vi "Deep Copy.vi"(7 "Tree ID":string, 8 "Error In":errorcluster, 11 "Tree Manager":T1) -> (0 "Error Out":errorcluster, 3 "Tree Manager":T1, 5 "Unique ID of Copied Tree":string)   [LabVIEW 2020, in "NI_VIAnCFGDataStructure.lvlib" / "Tree.lvclass"]
doc: "Deep copy of a Tree and its attributes. Copies the Children of the Tree all the way down. On all attributes that are Tree Data types a Copy method is invoked. Overwrite the Copy the method in child types of Tree Data to implement special copying mechanism. The Default mechanism is copying by values i.e. LV fork.\n\n<b>WARNING</b> Running this method on a big tree might result in a significantly slower operation than Shallow Copy method. Make sure you need to copy all the Children. If not use Shallow Copy method."
uses:
  <vilib>/addons/analyzer/VIAnCFGDataStructure/Tree Manager/Tree.lvclass
  <vilib>/addons/analyzer/VIAnCFGDataStructure/Tree Manager/Typedefs/Session Handle.ctl
  <vilib>/addons/analyzer/VIAnCFGDataStructure/Tree Manager/Tree.lvclass/Tree.ctl
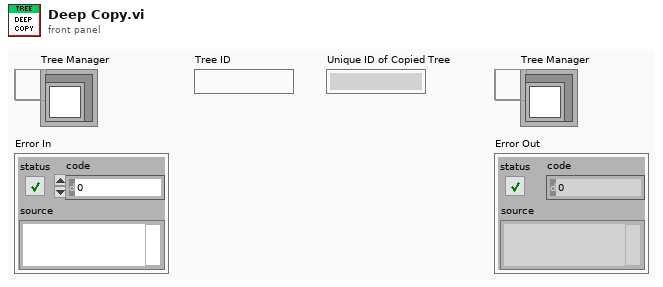
[diagram p1: front panel]
types:
  T1 = typedef "NI_VIAnCFGDataStructure.lvlib/Tree.lvclass/Session Handle.ctl" = refnum<data-value>
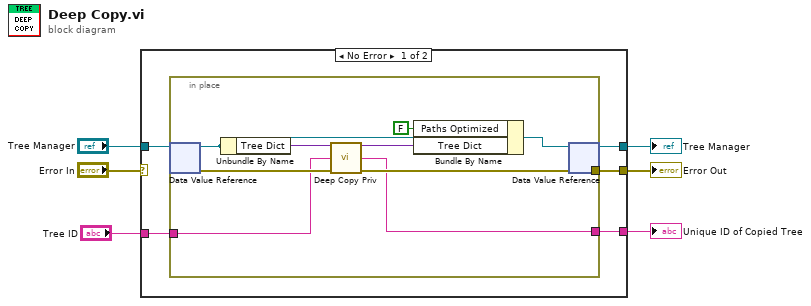
[diagram p0: block diagram]
diagram:
  n1 = case shown="No Error" "Error In" {
    selector: "Error In" -> [_ w21]
    tunnel: "Tree Manager" -> [w11 w22]
    tunnel: [w10 w22] -> w5
    tunnel: [w9 w21] -> w3
    tunnel: "Tree ID" -> [w8 _]
    tunnel: [w7 _] -> w1
    frame No Error {
      n2 = in-place {
        in-place-border: [w19] -> w9
        in-place-border: w8 -> [w16]
        in-place-border: [w15] -> w7
        n3 = in-place-dvr #1(w11) -> (w20:refnum<class "Tree.lvclass">, w17:errorcluster)
        n4 = Unbundle By Name(w20) -> ("Tree Dict"=w14:variant)
        n5 = call <vilib>:"Deep Copy Priv.vi"("Tree Dictionary In"=w14, "Unique ID"=w16, "error in"=w17) -> ("Tree Dictionary Out"=w13:variant, "ID"=w15:string, "error out"=w19:errorcluster)  [unwired: 10 in]
        n6 = Bundle By Name(cluster=w20, "Paths Optimized"=FALSE, "Tree Dict"=w13) -> (w18:refnum<class "Tree.lvclass">)
        n7 = in-place-dvr #1(w18) -> (w10:T1)  [unwired: 1 out]
      }
    }
    frame Error {
    }
  }
  "Tree Manager" <- w5
  "Error Out" <- w3
  "Unique ID of Copied Tree" <- w1
